vi "RealSense_HelloWorld_PointCloud Plus.vi"() -> ()   [LabVIEW 2023]
doc: "Simple Demo showing how to connect a RealSense Camera to stream COLOR and DEPTH from the stereo camera of a D4xx series camera. \n\nThis expands on the standard sample, by adding \n1. Subsampling for performance enhancement\n2. Collecting time-synched frames, and \n3. Option to remove texture from pointcloud"
uses:
  <vilib>/picture/3D Picture Control/NI_3D Picture Control.lvlib
  <vilib>/Utility/miscctls.llb/LV3DPointTypeDef.ctl
  <vilib>/Utility/miscctls.llb/LVRGBAColorTypeDef.ctl
  <vilib>/picture/3D Picture Control/Object/Create Object (name).vi
panel:
  in  "Display tab":T1(tab)=enum."Color + Depth"
  in  "Sync frames":T2(ring)
  out "Found \nRealSense":bool=TRUE
  out "height":i32=720
  out "width":i32=1280
  out "init results":T3={"camera name"="Intel RealSense 415", "camera S/N"="725112060291", "F/W"="05.08.09.00", "Sensor name"="Stereo Module", "api_version"=20800, "rscontext"=119411024, "device_list"=120905744, "device count"=2, "Dev out"=117239280, "sensor_list"=117821936, "sensor count"=2, "Sensor out"=325562496}
  in  "Select Resolution":u16(ring)=27 items=["424 x 240 @6fps", "424 x 240 @15fps", "424 x 240 @30fps", "424 x 240 @60fps", "424 x 240 @90fps", "480 x 270 @6fps", "480 x 270 @15fps", "480 x 270 @30fps", "480 x 270 @60fps", "480 x 270 @90fps", "640 x 360 @6fps", "640 x 360 @15fps", "640 x 360 @30fps", "640 x 360 @60fps", "640 x 360 @90fps", "640 x 480 @6fps", "640 x 480 @15fps", "640 x 480 @30fps", "640 x 480 @60fps", "640 x 480 @90fps", "848 x 480 @6fps", "848 x 480 @15fps", "848 x 480 @30fps", "848 x 480 @60fps", "848 x 480 @90fps", "1280 x 720 @6fps", "1280 x 720 @15fps", "1280 x 720 @30fps"]
  in  "Sensor index":i32
  in  "Device index":i32
  out "L-R Baseline, mm":sgl=54.83181
  out "fy":sgl=952.6064 format="%#_5g"
  out "fx":sgl=952.6064 format="%#_5g"
  out "ppy":sgl=370.69974 format="%#_5g"
  out "ppx":sgl=634.5728 format="%#_5g"
  in  "Exposure,us":sgl=33000.0
  in  "Autoexposure":bool=TRUE
  in  "Depth Presets":T4(ring)=enum."Face2"
  in  "Color Presets":T5(ring)=enum."DS410 (DS5a) 4"
  in  "Laser on/off":bool=TRUE
  in  "Gain(16-248)":sgl=16.0 min=16 max=248
  in  "Update Presets":bool
  in  "Laser \nPower (mW)":dbl(slide)=155.72448 min=0.0 max=360.0 scale=0.36..360.0
  in  "Range Scale":enum16{"200m", "100m", "60m", "6m", "2m", "1m"}(ring)=enum."6m"
  out "RGB image":picture
  out "Depth map":sgl[][](graph)
  out "3D Picture":refnum<vi>(3d-picture)
  in  "Texture":bool=TRUE
  in  "Time average parameters":T6={"alphaT"=0.3, "deltaDispT(1/32 disp)"=20.0}
  in  "Time Filter":bool=TRUE
  in  "Spatial filter parameters":T7={"alphaXY"=0.5, "deltaDispXY (1/32 disp)"=20.0, "iterations"=2} {"iterations" min=1 max=8; "deltaDispXY (1/32 disp)" min=0.001 max=65000; "alphaXY" min=0.001 max=1}
  in  "Spatial Filter":bool=TRUE
  in  "Persist":bool=TRUE
  out "init error":string="No Error\rNo Error\rNo Error\rNo Error\rNo Error\rNo Error\rNo Error\rNo Error\rNo Error\rNo Error\rNo Error"
  out "Start Error":string="No Error\rNo Error\rNo Error"
  out "Config error":string="No Error\rNo Error"
  out "Close Error":string="No Error\rNo Error\rNo Error\rNo Error"
  out "Time stamp, ms":dbl format="%_10f"
  out "Frame number":u64
  out "Time stamp 2, ms":dbl format="%_10f"
  out "Frame number 2":u64
  out "Timestamp domain":u16(ring) items=["Hardware clock", "System Time", "Count"]
  out "Timestamp domain 2":u16(ring) items=["Hardware clock", "System Time", "Count"]
  out "iteration":i32=357
  in  "stop":bool=TRUE
  # "RealSense Hello World: PointCloud + Post Process"
  # "This demo shows how to connect a RealSense D4xx Stereo Depth Camera, and display the textured PointCloud."
  # "Note; When you change Depth Preset you need to stop and restart for the HDAD settings to take effect.\n\nTry the Color preset called \"Remove IR2\". It will remove the laser projector from the RGB 1280x720 image."
  # "INTRINSICS & EXTRINSICS"
  # "SELECT THE RESOLUTION"
  # "DEPTH MAP"
  # "COLOR"
  # "Changes Color scale for Depth Map."
  # "20-1660000"
  # "3D POINTCLOUD"
  # "Rotate: Drag image\nMove X-Y: HOLD DOWN CTRL while dragging.\nZoom: SHIFT while dragging."
  # "POST PROCESS"
  # "ON\n\nOFF"
  # "Restart to take effect"
  # "Alph can have values from 0 to 1\n1 is zero filtering, and 0 is max filtering."
  # "ERRORS"
  # "If you do not see the Hardware clock then you will need to apply \nWindows fix. See diagram."
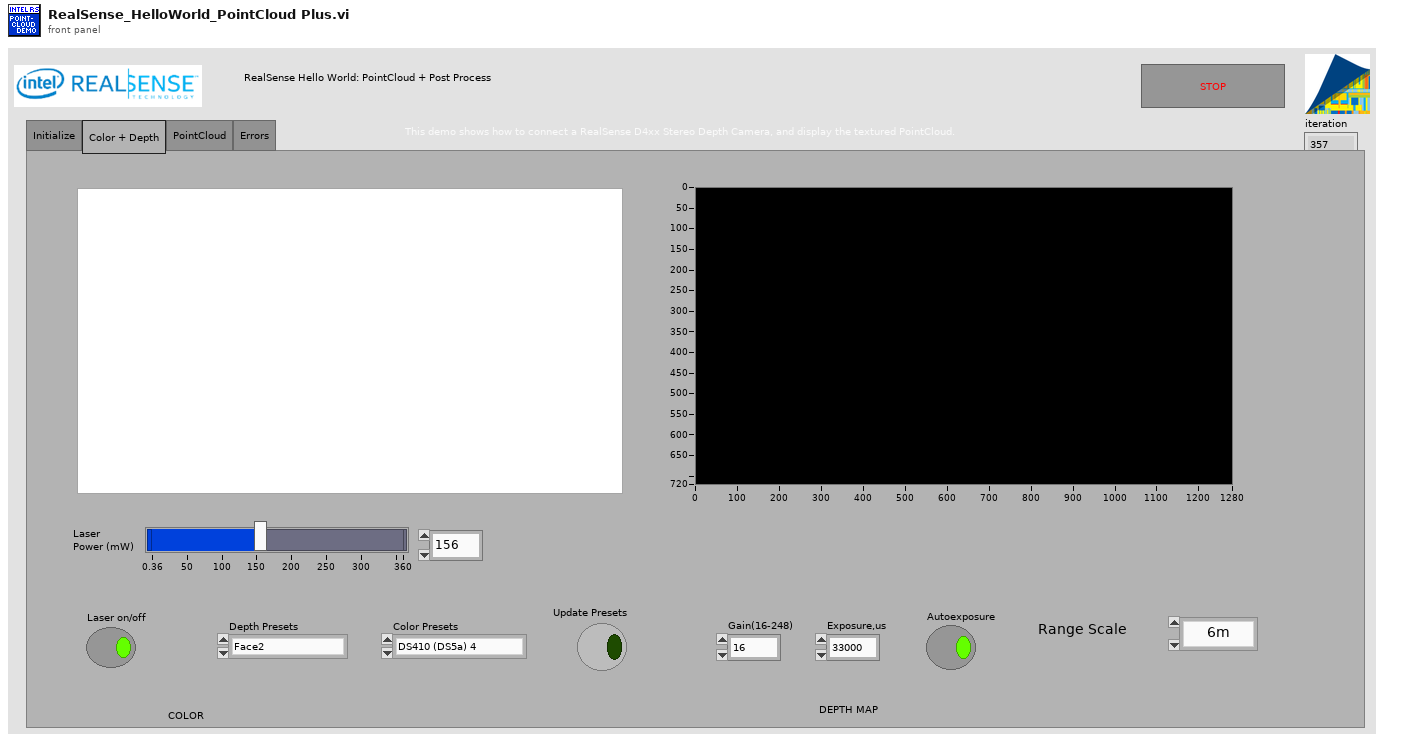
[diagram p1: front panel]
types:
  T1 = enum32{"Initialize", "Color + Depth", "PointCloud", "Errors"}
  T2 = enum16{"Sync on timestamp", "Sync on frame counter"}
  T3 = cluster{"camera name":string, "camera S/N":string, "F/W":string, "Sensor name":string, "api_version":i32, "rscontext":u64, "device_list":u64, "device count":i32, "Dev out":u64, "sensor_list":u64, "sensor count":i32, "Sensor out":u64}
  T4 = enum16{"Custom", "Original", "New Depth 1", "New Depth 2", "Depth Active 1", "Active 3D Scan", "Active Short A", "Active Short C", "Face", "Face2", "Best Box", "High Density", "Medium Density", "High Accuracy", "Hand", "Short Range", "Flat wall", "Load .JSON", "Load .JSON2"}
  T5 = enum16{"Custom", "RS400 (DS5p)", "RS400 (DS5p) 2", "RS400 (DS5p) 3", "RS400 (DS5p) 4", "RS400 (DS5p) 5", "RS410 (DS5a)", "RS410 (DS5a) 2", "DS410 (DS5a) 3", "DS410 (DS5a) 4", "DS410+IR", "DS5LR", "DS5LR-2", "DS5LR no pattern", "RS410 Remove IR", "RS410 Remove IR 2", "DS5micro", "D435"}
  T6 = cluster{"alphaT":sgl, "deltaDispT(1/32 disp)":sgl}
  T7 = cluster{"alphaXY":sgl, "deltaDispXY (1/32 disp)":sgl, "iterations":i32}
  T8 = cluster{"width":i32, "height":i32, "fps":i32, "Profile":u64, "ppx":sgl, "ppy":sgl, "fx":sgl, "fy":sgl, "model":u32}
  T9 = cluster{"Stream type":enum16{"Depth", "Color (ext.)", "Color (left) ", "IR Left", "IR Right", "IR Left (Y16)", "IR Right (Y16)"}, "frame out":u64, "width":i32, "height":i32, "Time stamp":dbl, "Frame number":u64}
  T10 = cluster{"focal length (pixels)":sgl, "baseline, mm":sgl, "z_units":sgl, "Y height":i32, "X width":i32, "Scale":i32, "Color format":enum16{"Monochrome", "RGB internal (RGB)"}}
  T11 = enum16{"Points", "Lines", "Line Strip", "Line Loop", "Triangles", "Triangle Strip", "Triangle Fan", "Quads", "Quad Strip", "Polygon"}
  T12 = enum16{"Overall", "Per Primitive", "Per Vertex", "Binding Off"}
  T13 = typedef "LVRGBAColorTypeDef.ctl" = cluster{"Red":sgl, "Green":sgl, "Blue":sgl, "Alpha":sgl}
  T14 = enum16{"Depth", "Color (ext.)", "Color (left) ", "IR Left", "IR Right", "IR Left (Y16)", "IR Right (Y16)"}
  T15 = cluster{"R":dbl, "G":dbl, "B":dbl, "Alpha":dbl}[]
  T16 = typedef "LV3DPointTypeDef.ctl" = cluster{"X":sgl, "Y":sgl, "Z":sgl}
  T17 = cluster{"Alpha":sgl, "Blue":sgl, "Green":sgl, "Red":sgl}
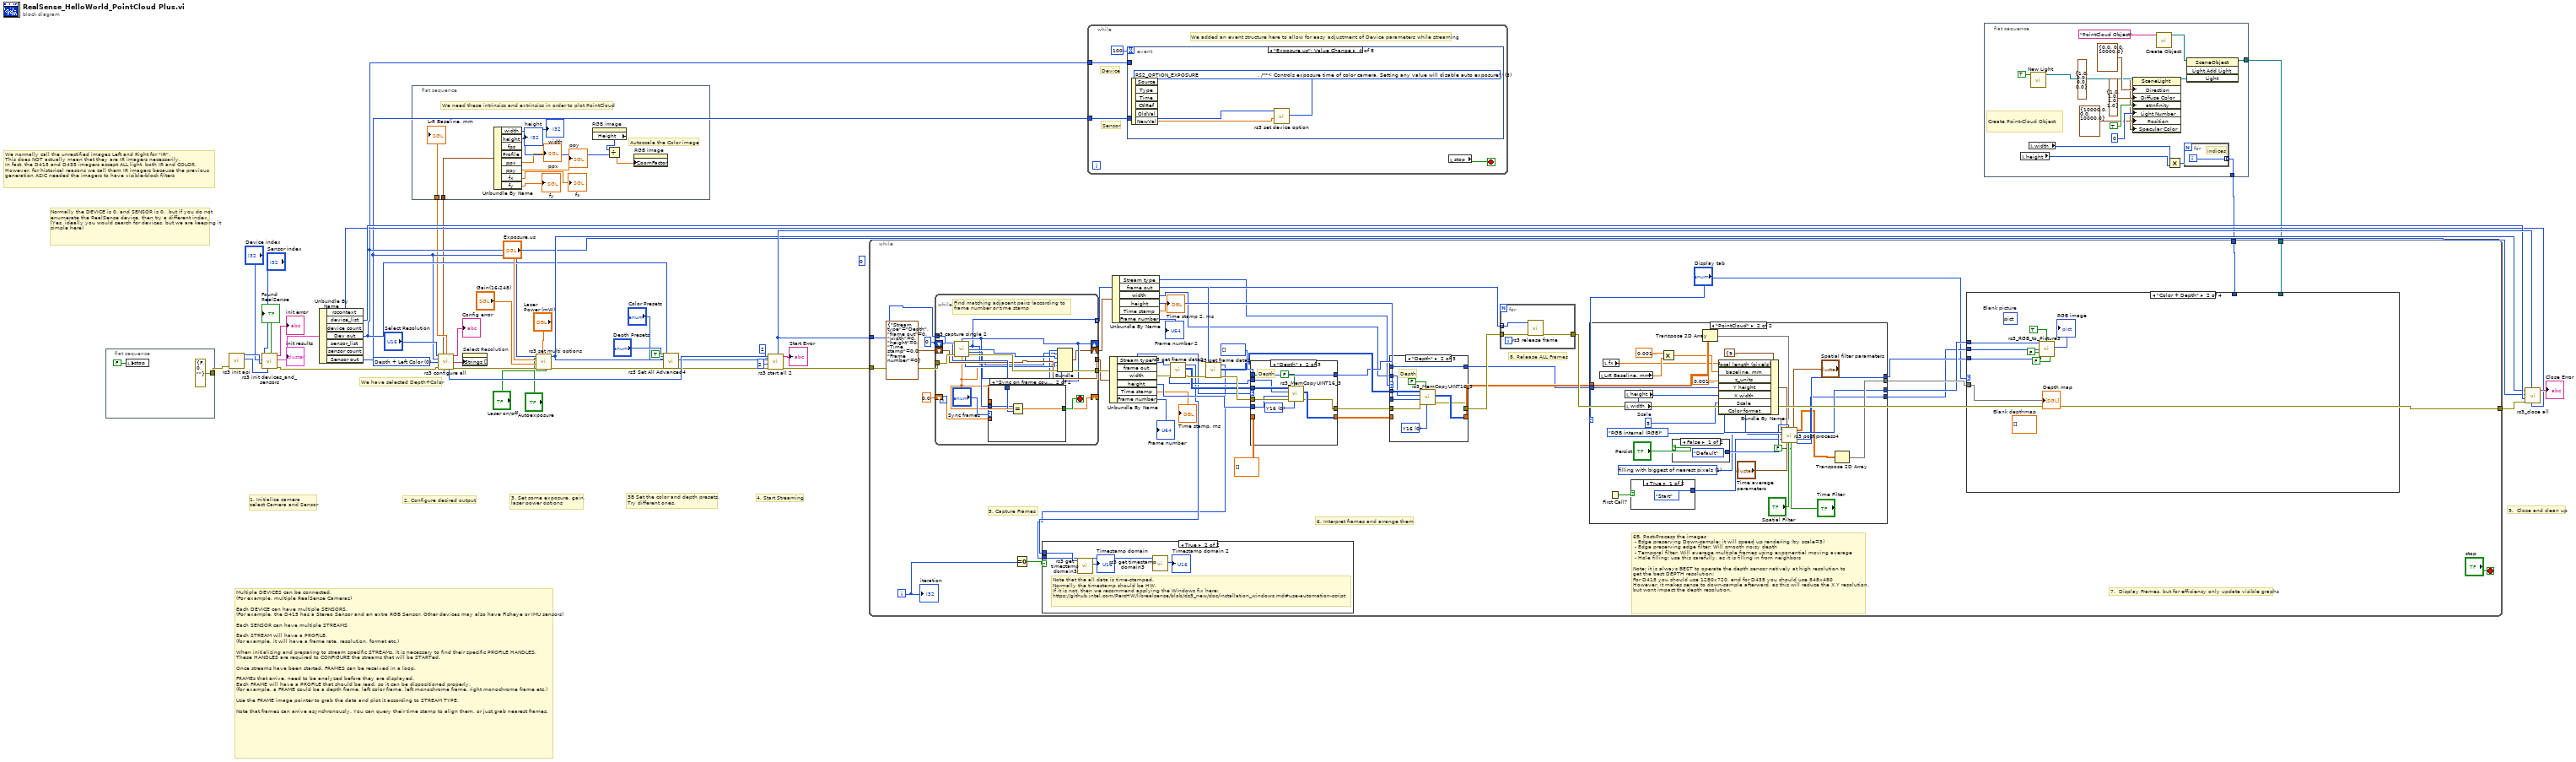
[diagram p0: block diagram]
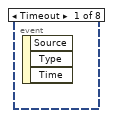
[diagram p2: hidden frame]
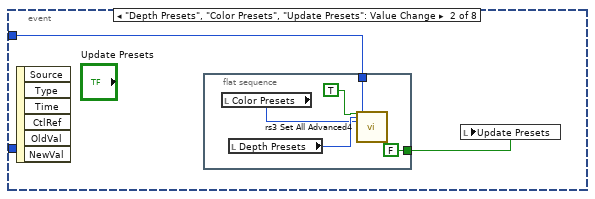
[diagram p3: hidden frame]
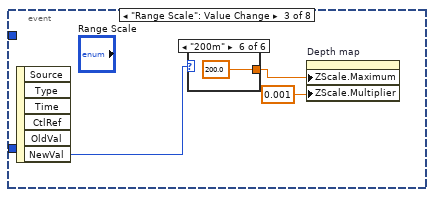
[diagram p4: hidden frame]
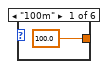
[diagram p5: hidden frame]
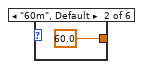
[diagram p6: hidden frame]
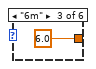
[diagram p7: hidden frame]
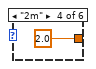
[diagram p8: hidden frame]
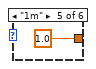
[diagram p9: hidden frame]
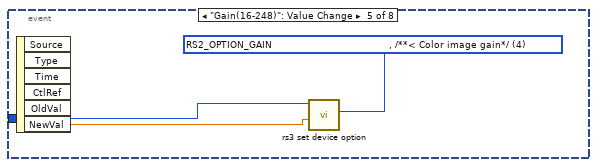
[diagram p10: hidden frame]
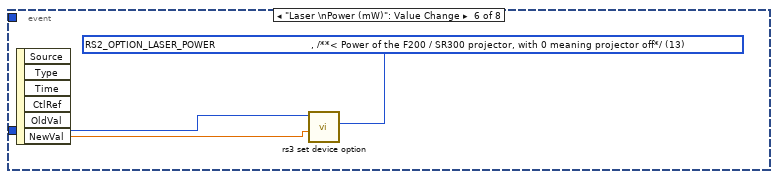
[diagram p11: hidden frame]
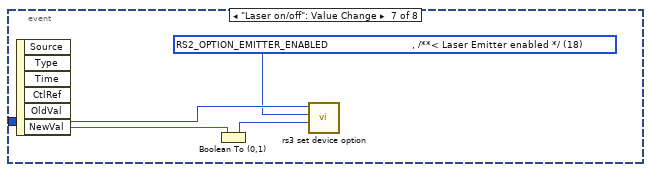
[diagram p12: hidden frame]
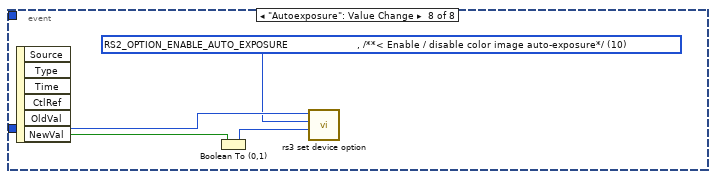
[diagram p13: hidden frame]
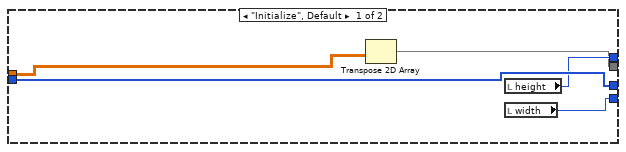
[diagram p14: hidden frame]
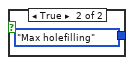
[diagram p15: hidden frame]
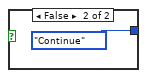
[diagram p16: hidden frame]
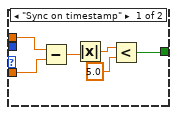
[diagram p18: hidden frame]
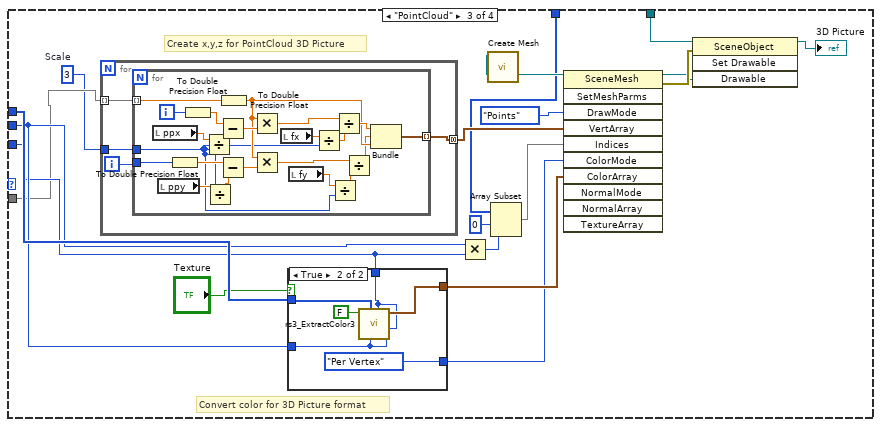
[diagram p20: hidden frame]
diagram:
  (unwired) 0 ("Decimate")
  w29 = u16 0 items=["Depth + Left Color", "Unrectified L + R", "Rectified L + R"] ("Stream selection")
  # "3B Set the color and depth presets.\nTry different ones."
  # "We normally call the unrectified images Left and Right for \"IR\". \nThis does NOT actually mean that they are IR imagers necessarily. \nIn fact, the D415 and D435 imagers accept ALL light, both IR and COLOR.\nHowever, for historical reasons we call them IR imagers because the previous generation ASIC needed the imagers to have visible-block filters"
  # "We have selected Depth+Color"
  # "Normally the DEVICE is 0, and SENSOR is 0,  but if you do not enumerate the RealSense device, then try a different index.\n(Yes, ideally you would search for devices, but we are keeping it simple here)"
  # "Multiple DEVICES can be connected. \n(For example, multiple RealSense Cameras)\n\nEach DEVICE can have multiple SENSORS. \n(For example, the D415 has a Stereo Sensor and an extra RGB Sensor. Other devices may also have Fisheye or IMU sensors) \n\nEach SENSOR can have multiple STREAMS\n\nEach STREAM will have a PROFILE. \n(for example, it will have a frame rate, resolution, format etc.)\n\nWhen initializing and preparing to stream specific STREAMs, it is necessary to find their specific PROFILE HANDLES.\nThese HANDLES are required to CONFIGURE the streams that will be STARTed. \n\nOnce streams have been started, FRAMES can be received in a loop. \n \nFRAMEs that arrive, need to be analyzed before they are displayed. \nEach FRAME will have a PROFILE that should be read, so it can be dispositioned properly.\n(for example, a FRAME could be a depth frame, left color frame, left monochrome frame, right monochrome frame etc.)\n\nUse the FRAME image pointer to grab the data and plot it according to STREAM TYPE.\n\nNote that frames can arrive asynchronously. You can query their time stamp to align them, or just grab nearest frames."
  # "9.  Close and clean up"
  # "4. Start Streaming"
  # "3. Set some exposure, gain, \nlaser power options"
  # "2. Configure desired output"
  # "1. Initialize camera\nselect Camera and Sensor"
  n1 = flat-sequence {
    tunnel: [errorcluster {"status"=FALSE, "code"=0, "source"=""} ("error in")] -> w30
    frame #0 {
      n2 = local write "stop"(FALSE ("stop")) -> ()
    }
  }
  n3 = call "rs3 init api.vi"("error in (no error)"=w30) -> ("rscontext"=w9:u64, "api_version"=w10:i32)  [unwired: 8 in, 1 out]
  n4 = call "rs3 init devices_and_sensors.vi"("rscontext"=w9, "api_version"=w10, "Select Device"="Device index", "Select Sensor"="Sensor index") -> ("error out"=w6:errorcluster, "init results"=w4:T3, "init error"=→"init error":string, "Found RealSense"=→"Found \nRealSense":bool)  [unwired: 1 in, 3 out]
  "init results" <- w4
  n5 = Unbundle By Name(w4) -> ("rscontext"=w35:u64, "device_list"=w36:u64, "Dev out"=w17:u64, "Sensor out"=w16:u64)  [unwired: 3 out]
  n6 = flat-sequence {
    tunnel: w14 -> [w53]
    tunnel: w13 -> [w52]
    frame #0 {
      # "Autoscale the Color image"
      # "We need these intrinsics and extrinsics in order to plot PointCloud"
      n7 = Unbundle By Name(w52) -> ("width"=→"width":i32, "height"=w50:i32, "ppx"=→"ppx":sgl, "ppy"=→"ppy":sgl, "fx"=→"fx":sgl, "fy"=→"fy":sgl)  [unwired: 2 out]
      "height" <- w50
      n8 = property on="RGB image" class="Pict"() -> ("Height"=w51:u32)  [unwired: 2 in, 2 out]
      n9 = Divide(x=w51, y=w50) -> (x/y=w49:dbl)
      n10 = property on="RGB image" class="Pict"("ZoomFactor"=w49) -> ()  [unwired: 2 in, 2 out]
      "L-R Baseline, mm" <- w53
    }
  }
  n11 = call "rs3 configure all.vi"("Select Resolution"="Select Resolution", "Sensor in"=w16, "Stream selection"=w29, "error in (no error)"=w6) -> ("Output stream L"=w13:T8, "config error"=→"Config error":string, "Output stream"=w31:string[], "L-R Baseline, mm"=w14:sgl, "Stream Profile Handles"=w41:u64[], "error out"=w28:errorcluster)  [unwired: 2 in, 4 out]
  n12 = property on="Select Resolution" class="Ring (strict)"("Strings []"=w31) -> ()  [unwired: 2 in, 2 out]
  n13 = call "rs3 set multi options.vi"("laser on/off"="Laser on/off", "autoexposure"="Autoexposure", "Laser power, mW (0-360)"="Laser \nPower (mW)", "error in (no error)"=w28, "Gain(16-248)"="Gain(16-248)", "Exposure, us"="Exposure,us", "Sensor in"=w16) -> ("error out"=w22:errorcluster, "Sensor out"=w27:u64)  [unwired: 2 in, 1 out]
  n14 = call "rs3 Set All Advanced4.vi"("Set Color Corr"=TRUE, "Depth Presets"="Depth Presets", "Color Presets"="Color Presets", "error in (no error)"=w22, "device in"=w17) -> ("error out"=w21:errorcluster)  [unwired: 20 in, 2 out]
  n15 = call "rs3 start all 2.vi"("capacity"=2, "error in (no error)"=w21, "Count of Streams"=2, "Sensor in"=w27, "Stream profile array"=w41) -> ("error out"=w32:errorcluster, "Config Error"=→"Start Error":string, "queue out"=w40:u64)  [unwired: 3 in, 1 out]
  n16 = while {
    tunnel: w40 -> [w94]
    tunnel: w32 -> [w93]
    tunnel: [w73] -> w39
    tunnel: w12 -> [w96]
    tunnel: w11 -> [w95]
    i -> [w65]
    stop <- "stop" stop-if-true
    # "6B. Post-Process the images \n - Edge preserving Down-sample: it will speed up rendering (try scale=3)\n - Edge preserving edge filter: Will smooth noisy depth\n - Temporal filter: Will average multiple frames using exponential moving average\n - Hole filling: use this carefully, as it is filling in from neighbors\n\nNote: it is always BEST to operate the depth sensor natively at high resolution to \nget the best DEPTH resolution: \nFor D415 you should use 1280x720, and for D435 you should use 848x480\nHowever, it makes sense to down-sample afterward, as this will reduce the X,Y resolution, \nbut wont impact the depth resolution."
    # "8. Release ALL Frames"
    # "7.  Display Frames, but for efficiency only update visible graphs"
    # "6. Interpret frames and arrange them"
    # "5. Capture Frames"
    n17 = while {
      tunnel: w94 -> [w159]
      tunnel: [w158] -> w91
      tunnel: w93 -> [w157]
      shift-right: [w150] -> _
      shift-left: u64 0 ("Frame number") -> [w155]
      shift-right: [w149] -> w87
      shift-left: T9 {"Stream type"=enum."Depth", "frame out"=0, "width"=0, "height"=0, "Time stamp"=0.0, "Frame number"=0} -> [w154]
      tunnel: [w154] -> w88
      tunnel: [w148] -> w75 mode=indexing
      shift-right: [w145] -> _
      shift-left: 0.0 ("Time stamp") -> [w146]
      stop <- w156 stop-if-true
      # "Find matching adjacent pairs (according to frame number or time stamp"
      n18 = call "rs3 capture single 2.vi"("queue in"=w159, "error in (no error)"=w157) -> ("Frame number"=w150:u64, "frame out"=w148:u64, "width"=w153:i32, "Stream type"=w151:T14, "Time stamp"=w145:dbl, "height"=w152:i32, "error out"=w158:errorcluster)  [unwired: 3 in, 4 out]
      n19 = case shown="\"Sync on frame counter\"" "Sync frames" {
        tunnel: [w163 w168] -> w156
        tunnel: w155 -> [_ w167]
        tunnel: w150 -> [_ w166]
        tunnel: w146 -> [w165 _]
        tunnel: w145 -> [w164 _]
        frame "Sync on timestamp" {
          n20 = Subtract(x=w164, y=w165) -> (x-y=w162:dbl)
          n21 = Absolute Value(x=w162) -> (abs(x)=w161:dbl)
          n22 = Less?(x=w161, y=5.0) -> (x < y?=w163:bool)
        }
        frame "Sync on frame counter" {
          n23 = Equal?(x=w166, y=w167) -> (x = y?=w168:bool)
        }
      }
      n24 = Bundle("Stream type"=w151, "frame out"=w148, "width"=w153, "height"=w152, "Time stamp"=w145, "Frame number"=w150) -> (w149:T9)  [unwired: 1 in]
    }
    n25 = Equal To 0?(x=w65) -> (x = 0?=w55:bool)
    n26 = Unbundle By Name(w88) -> ("Stream type"=w76:T14, "frame out"=w89:u64, "width"=w78:i32, "height"=w77:i32, "Time stamp"=→"Time stamp, ms":dbl, "Frame number"=→"Frame number":u64)
    n27 = Unbundle By Name(w87) -> ("Stream type"=w57:T14, "frame out"=w86:u64, "width"=w56:i32, "height"=w58:i32, "Time stamp"=→"Time stamp 2, ms":dbl, "Frame number"=→"Frame number 2":u64)
    n28 = call "rs3 get frame data2.vi"("error in (no error)"=w91, "device in"=w89) -> ("error out"=w90:errorcluster, "2D Depth Output"=w81:u16[][], "device out"=w67:u64)  [unwired: 6 in, 1 out]
    n29 = call "rs3 get frame data2.vi"("error in (no error)"=w90, "device in"=w86) -> ("error out"=w83:errorcluster, "2D Depth Output"=w80:u16[][], "device out"=w66:u64)  [unwired: 6 in, 1 out]
    n30 = case shown="True" w55 {
      tunnel: w67 -> [_ w141]
      tunnel: w66 -> [_ w140]
      frame False {
      }
      frame True {
        # "Note that the all data is time-stamped. \nNormally the timestamp should be HW. \nIf it is not, then we recommend applying the Windows fix here:\nhttps://github.intel.com/PercHW/librealsense/blob/ds5_new/doc/installation_windows.md#use-automation-script"
        n31 = call "rs3 get timestamp domain3.vi"("frame in"=w141) -> ("Timestamp domain"=→"Timestamp domain":u16)  [unwired: 7 in, 3 out]
        n32 = call "rs3 get timestamp domain3.vi"("frame in"=w140) -> ("Timestamp domain"=→"Timestamp domain 2":u16)  [unwired: 7 in, 3 out]
      }
    }
    n33 = case shown="\"Depth\"" w76 {
      tunnel: [w250 w259 w268] -> w98
      tunnel: [w252 w260 w266] -> w97
      tunnel: sgl[][] [] ("2D Array Output") -> [w252 _ w266]
      tunnel: u8[] [] ("Output Array") -> [w251 w258 _]
      tunnel: [w251 w258 w267] -> w79
      tunnel: w83 -> [w250 w257 w262]
      tunnel: w81 -> [_ w256 w265]
      tunnel: w78 -> [_ w255 w264]
      tunnel: w77 -> [_ w254 w263]
      frame "Color (ext.)", Default {
      }
      frame "Depth" {
        w261 = u16 0 items=["Y16", "Y8"] ("Image format")
        # "Depth"
        n34 = call "rs3_MemCopyUINT16_3.vi"("Image format"=w261, "Transpose"=FALSE, "error in (no error)"=w257, "Height"=w254, "Width"=w255, "Zimage pointer"=w256) -> ("error out"=w259:errorcluster, "2D Array Output"=w260:u16[][])  [unwired: 4 in]
      }
      frame "Color (left) " {
        # "Color"
        n35 = call "rs3_MemCopyRGB_IR.vi"("Zimage pointer"=w265, "RGB  X, width"=w264, "RGB Y, height"=w263, "Monochrome(T)/Color(F)"=FALSE ("Grey(T)/Color(F)"), "error in (no error)"=w262) -> ("Output Array"=w267:u8[], "error out"=w268:errorcluster)  [unwired: 9 in]
      }
    }
    n36 = case shown="\"Depth\"" w57 {
      tunnel: [w232 w238 w247] -> w74
      tunnel: w98 -> [w232 w239 w248]
      tunnel: w97 -> [w231 _ w245]
      tunnel: [w231 w240 w245] -> w64
      tunnel: [w230 w241 w246] -> w63
      tunnel: w79 -> [w230 w241 _]
      tunnel: w80 -> [_ w236 w244]
      tunnel: w56 -> [_ w235 w242]
      tunnel: w58 -> [_ w234 w243]
      frame "Color (ext.)", Default {
      }
      frame "Depth" {
        w237 = u16 0 items=["Y16", "Y8"] ("Image format")
        # "Depth"
        n37 = call "rs3_MemCopyUINT16_3.vi"("Image format"=w237, "Transpose"=FALSE, "error in (no error)"=w239, "Height"=w234, "Width"=w235, "Zimage pointer"=w236) -> ("error out"=w238:errorcluster, "2D Array Output"=w240:u16[][])  [unwired: 4 in]
      }
      frame "Color (left) " {
        # "Color"
        n38 = call "rs3_MemCopyRGB_IR.vi"("Zimage pointer"=w244, "RGB  X, width"=w242, "RGB Y, height"=w243, "Monochrome(T)/Color(F)"=FALSE ("Grey(T)/Color(F)"), "error in (no error)"=w248) -> ("Output Array"=w246:u8[], "error out"=w247:errorcluster)  [unwired: 9 in]
      }
    }
    n39 = for {
      tunnel: w75 -> [w144] mode=indexing
      tunnel: w74 -> [w143]
      tunnel: [w142] -> w73
      n40 = call "rs3 release frame.vi"("error in (no error)"=w143, "Device"=w144) -> ("error out"=w142:errorcluster)  [unwired: 7 in, 2 out]
    }
    n41 = case shown="\"PointCloud\"" "Display tab" {
      tunnel: w64 -> [w101 w133]
      tunnel: w63 -> [w104 w132]
      tunnel: [w100 w131] -> w62
      tunnel: [w104 w130] -> w61
      tunnel: [w103 w129] -> w60
      tunnel: [w102 w128] -> w59
      frame "Initialize", Default {
        n42 = Transpose 2D Array(2D array=w101) -> (transposed array=w100:sgl[][])
        n43 = local read "height"() -> (w103:i32)
        n44 = local read "width"() -> (w102:i32)
      }
      frame "PointCloud" {
        w115 = 1 items=["filling with left pixel", "filling with biggest of nearest pixels", "filling with smallest of nearest pixels"] ("hole fill algo")
        w127 = 3  # Scale
        n45 = local read "L-R Baseline, mm"() -> (w113:sgl)
        n46 = local read "fx"() -> (w111:sgl)
        n47 = First Call?() -> (First Call?: T/F=w108:bool)
        n48 = local read "height"() -> (w118:i32)
        n49 = local read "width"() -> (w117:i32)
        n50 = case shown="True" w108 {
          tunnel: [enum16{"Start", "Continue", "End", "Do Nothing"}."Start" ("Algo step") enum16{"Start", "Continue", "End", "Do Nothing"}."Continue" ("Algo step")] -> w107
          frame True {
          }
          frame False {
          }
        }
        n51 = Multiply(x=sgl 0.001 ("z_units"), y=w113) -> (x*y=w112:sgl)
        n52 = case shown="False" "Persist" {
          tunnel: [enum16{"Custom", "Default", "Max holefilling"}."Default" ("Temporal persistence \nHole-filling") enum16{"Custom", "Default", "Max holefilling"}."Max holefilling" ("Temporal persistence \nHole-filling")] -> w125
          frame False {
          }
          frame True {
          }
        }
        n53 = Transpose 2D Array(2D array=w133) -> (transposed array=w110:sgl[][])
        n54 = Bundle By Name(cluster=T10 {"focal length (pixels)"=961.0, "baseline, mm"=0.015000001, "z_units"=0.001, "Y height"=720, "X width"=1280, "Scale"=3, "Color format"=enum."RGB internal (RGB)"} ("downsample  parameters"), "focal length (pixels)"=w111, "baseline, mm"=w112, "z_units"=sgl 0.001, "Y height"=w118, "X width"=w117, "Scale"=w127, "Color format"=enum16{"Monochrome", "RGB internal (RGB)"}."RGB internal (RGB)") -> (w120:T10)
        n55 = call "rs3 post process4.vi"("Depth Input"=w110, "Color input"=w132, "hole fill algo"=w115, "Algo step"=w107, "downsample  parameters"=w120, "Time average parameters"="Time average parameters", "Temporal persistence \nHole-filling"=w125, "Spatial Filter"="Spatial Filter", "Time Filter"="Time Filter", "Holefill"=FALSE, "Spatial filter parameters"="Spatial filter parameters") -> ("Depth Output"=w109:sgl[][], "Color output"=w130:u8[], "output width"=w128:i32, "output height"=w129:i32)  [unwired: 4 in, 1 out]
        n56 = Transpose 2D Array(2D array=w109) -> (transposed array=w131:sgl[][])
      }
    }
    n57 = case shown="\"Color + Depth\"" "Display tab" {
      tunnel: w61 -> [_ w173 w195 _]
      tunnel: w62 -> [_ w172 w178 _]
      tunnel: w96 -> [_ _ w187 _]
      tunnel: w95 -> [_ _ w186 _]
      tunnel: w59 -> [_ w171 w180 _]
      tunnel: w60 -> [_ w170 w179 _]
      frame "Initialize", Default {
      }
      frame "Color + Depth" {
        (unwired) sgl[][] []  # Blank depthmap
        (unwired) picture bytes[33]  # Blank picture
        n58 = call "rs3_RGB_to_Picture3.vi"("RGB array"=w173, "Color(T)/Greyscale(F)"=TRUE, "RGB  X, width"=w171, "RGB Y, height"=w170, "AWB"=FALSE, "White Balance"=FALSE) -> ("new picture"=→"RGB image":picture)  [unwired: 8 in, 1 out]
        "Depth map" <- w172
      }
      frame "PointCloud" {
        w177 = 3  # Scale
        # "Convert color for 3D Picture format"
        # "Create x,y,z for PointCloud 3D Picture"
        n59 = for {
          tunnel: w178 -> [w207] mode=indexing
          tunnel: [w206] -> w190 mode=concatenating
          tunnel: w177 -> [w204]
          i -> [w205]
          n60 = for {
            tunnel: w207 -> [w229] mode=indexing
            tunnel: w205 -> [w228]
            tunnel: [w227] -> w206 mode=indexing
            tunnel: w204 -> [w208]
            i -> [w226]
            n61 = local read "ppx"() -> (w216:sgl)
            n62 = local read "ppy"() -> (w214:sgl)
            n63 = To Double Precision Float(number=w228) -> (double precision float=w220:dbl)
            n64 = To Double Precision Float(number=w226) -> (double precision float=w222:dbl)
            n65 = Divide(x=w216, y=w208) -> (x/y=w215:sgl)
            n66 = Divide(x=w214, y=w208) -> (x/y=w213:sgl)
            n67 = Subtract(x=w222, y=w215) -> (x-y=w221:dbl)
            n68 = Subtract(x=w220, y=w213) -> (x-y=w219:dbl)
            n69 = To Double Precision Float(number=w229) -> (double precision float=w218:dbl)
            n70 = Multiply(x=w218, y=w221) -> (x*y=w225:dbl)
            n71 = Multiply(x=w218, y=w219) -> (x*y=w223:dbl)
            n72 = local read "fx"() -> (w212:sgl)
            n73 = local read "fy"() -> (w210:sgl)
            n74 = Divide(x=w212, y=w208) -> (x/y=w211:sgl)
            n75 = Divide(x=w210, y=w208) -> (x/y=w209:sgl)
            n76 = Divide(x=w225, y=w211) -> (x/y=w224:dbl)
            n77 = Divide(x=w223, y=w209) -> (x/y=w217:dbl)
            n78 = Bundle(w224, w217, w218) -> (w227:cluster{dbl, dbl, dbl})  [unwired: 1 in]
          }
        }
        n79 = case shown="True" "Texture" {
          tunnel: w195 -> [_ w203]
          tunnel: [T13[] [{"Red"=1.0, "Green"=1.0, "Blue"=1.0, "Alpha"=0.0}] ("Color Array") w201] -> w189
          tunnel: [T12."Overall" ("Color Binding Mode") T12."Per Vertex" ("Color Binding Mode")] -> w182
          tunnel: w179 -> [_ w198]
          tunnel: w180 -> [_ w199]
          frame False {
          }
          frame True {
            n80 = call "rs3_ExtractColor3.vi"("Depth X"=w199, "Depth Y"=w198, "RGB Y"=w198, "RGB  X"=w199, "24bit Color Array"=w203, "White Balance"=FALSE) -> ("Norm Mesh Color"=w201:T15)  [unwired: 5 in]
          }
        }
        n81 = Multiply(x=w180, y=w179) -> (x*y=w183:i32)
        n82 = call <vilib>:"Create Mesh.vi"() -> ("New Mesh Refnum"=w192:refnum<vi>)  [unwired: 10 in, 1 out]
        n83 = Array Subset(array=w186, index=0, length=w183) -> (w185:i32[])
        n84 = invoke class="SceneMesh" method="SetMeshParms"(reference=w192, "DrawMode"=T11."Points" ("Draw Mode"), "VertArray"=w190, "Indices"=w185, "ColorMode"=w182, "ColorArray"=w189) -> (reference out=w193:refnum<vi>, error out=w194:errorcluster)  [unwired: 5 in, 9 out]
        n85 = invoke class="SceneObject" method="Set Drawable"(reference=w187, error in=w194, "Drawable"=w193) -> (reference out=→"3D Picture":refnum<vi>)  [unwired: 1 in, 3 out]
      }
      frame "Errors" {
      }
    }
    "iteration" <- w65
  }
  n86 = while {
    tunnel: w17 -> [w272]
    tunnel: w16 -> [w271]
    stop <- w273 stop-if-true
    # "Sensor"
    # "Device"
    # "We added an event structure here to allow for easy adjustment of Device parameters while streaming"
    n87 = event shown="[3] \"Exposure,us\": Value Change" {
      selector: _ -> [_ _ _ _ _ _ _ _]
      dyn-events: _ -> [_ _ _ _ _ _ _ _]
      timeout: 100 -> [_ _ _ _ _ _ _ _]
      tunnel: w272 -> [_ w275 _ _ _ _ _ _]
      tunnel: w271 -> [_ _ _ w292 w295 w298 w302 w306]
      event Timeout {
        n88 = event-data() -> ()  [unwired: 1 in, 3 out]
      }
      event "Depth Presets", "Color Presets", "Update Presets": Value Change {
        n89 = event-data() -> ()  [unwired: 1 in, 6 out]
        n90 = flat-sequence {
          tunnel: w275 -> [w277]
          tunnel: [FALSE ("Update Presets")] -> w274
          frame #0 {
            n91 = local read "Color Presets"() -> (w279:T5)
            n92 = local read "Depth Presets"() -> (w280:T4)
            n93 = call "rs3 Set All Advanced4.vi"("Set Color Corr"=TRUE, "Depth Presets"=w280, "Color Presets"=w279, "device in"=w277) -> ()  [unwired: 21 in, 3 out]
          }
        }
        n94 = local write "Update Presets"(w274) -> ()
      }
      event "Range Scale": Value Change {
        n95 = event-data() -> ("NewVal"=w282:enum16{"200m", "100m", "60m", "6m", "2m", "1m"})  [unwired: 1 in, 5 out]
        n96 = case shown="\"200m\"" w282 {
          tunnel: [100.0 ("Z Scale.Offset and Multiplier:Multiplier") 60.0 ("Z Scale.Offset and Multiplier:Multiplier") 6.0 ("Z Scale.Offset and Multiplier:Multiplier") 2.0 ("Z Scale.Offset and Multiplier:Multiplier") 1.0 ("Z Scale.Offset and Multiplier:Multiplier") 200.0 ("Z Scale.Offset and Multiplier:Multiplier")] -> w281
          frame "100m" {
          }
          frame "60m", Default {
          }
          frame "6m" {
          }
          frame "2m" {
          }
          frame "1m" {
          }
          frame "200m" {
          }
        }
        n97 = property on="Depth map" class="IntGraph (strict)"("ZScale.Maximum"=w281, "ZScale.Multiplier"=0.001 ("Z Scale.Offset and Multiplier:Multiplier")) -> ()  [unwired: 2 in, 2 out]
      }
      event "Exposure,us": Value Change {
        w290 = u16 3 items=["    RS2_OPTION_BACKLIGHT_COMPENSATION                     , /**< Enable / disable color backlight compensation*/", "    RS2_OPTION_BRIGHTNESS                                 , /**< Color image brightness*/", "    RS2_OPTION_CONTRAST                                   , /**< Color image contrast*/", "    RS2_OPTION_EXPOSURE                                   , /**< Controls exposure time of color camera. Setting any value will disable auto exposure*/", "    RS2_OPTION_GAIN                                       , /**< Color image gain*/", "    RS2_OPTION_GAMMA                                      , /**< Color image gamma setting*/", "    RS2_OPTION_HUE                                        , /**< Color image hue*/", "    RS2_OPTION_SATURATION                                 , /**< Color image saturation setting*/", "    RS2_OPTION_SHARPNESS                                  , /**< Color image sharpness setting*/", "    RS2_OPTION_WHITE_BALANCE                              , /**< Controls white balance of color image. Setting any value will disable auto white balance*/", "    RS2_OPTION_ENABLE_AUTO_EXPOSURE                       , /**< Enable / disable color image auto-exposure*/", "    RS2_OPTION_ENABLE_AUTO_WHITE_BALANCE                  , /**< Enable / disable color image auto-white-balance*/", "    RS2_OPTION_VISUAL_PRESET                              , /**< Provide access to several recommend sets of option presets for the depth camera */", "    RS2_OPTION_LASER_POWER                                , /**< Power of the F200 / SR300 projector, with 0 meaning projector off*/", "    RS2_OPTION_ACCURACY                                   , /**< Set the number of patterns projected per frame. The higher the accuracy value the more patterns projected. Increasing the number of patterns help to achieve better accuracy. Note that this c", "    RS2_OPTION_MOTION_RANGE                               , /**< Motion vs. Range trade-off, with lower values allowing for better motion sensitivity and higher values allowing for better depth range*/", "    RS2_OPTION_FILTER_OPTION                              , /**< Set the filter to apply to each depth frame. Each one of the filter is optimized per the application requirements*/", "    RS2_OPTION_CONFIDENCE_THRESHOLD                       , /**< The confidence level threshold used by the Depth algorithm pipe to set whether a pixel will get a valid range or will be marked with invalid range*/", "    RS2_OPTION_EMITTER_ENABLED                            , /**< Laser Emitter enabled */", "    RS2_OPTION_FRAMES_QUEUE_SIZE                          , /**< Number of frames the user is allowed to keep per stream. Trying to hold-on to more frames will cause frame-drops.*/", "    RS2_OPTION_TOTAL_FRAME_DROPS                          , /**< Total number of detected frame drops from all streams */", "    RS2_OPTION_AUTO_EXPOSURE_MODE                         , /**< Auto-Exposure modes: Static, Anti-Flicker and Hybrid */", "    RS2_OPTION_POWER_LINE_FREQUENCY                       , /**< Power Line Frequency control for anti-flickering Off/50Hz/60Hz/Auto */", "    RS2_OPTION_ASIC_TEMPERATURE                           , /**< Current Asic Temperature */", "    RS2_OPTION_ERROR_POLLING_ENABLED                      , /**< disable error handling */", "    RS2_OPTION_PROJECTOR_TEMPERATURE                      , /**< Current Projector Temperature */", "    RS2_OPTION_OUTPUT_TRIGGER_ENABLED                     , /**< Enable / disable trigger to be outputed from the camera to any external device on every depth frame */", "    RS2_OPTION_MOTION_MODULE_TEMPERATURE                  , /**< Current Motion-Module Temperature */", "    RS2_OPTION_DEPTH_UNITS                                , /**< Number of meters represented by a single depth unit */", "    RS2_OPTION_ENABLE_MOTION_CORRECTION                   , /**< Enable/Disable automatic correction of the motion data */", "    RS2_OPTION_AUTO_EXPOSURE_PRIORITY                     , /**< Allows sensor to dynamically ajust the frame rate depending on lighting conditions */", "    RS2_OPTION_COUNT                                      , /**< Number of enumeration values. Not a valid input: intended to be used in for-loops. */"] ("RS Option")
        n98 = event-data() -> ("NewVal"=w291:sgl)  [unwired: 1 in, 5 out]
        n99 = call "rs3 set device option.vi"("value"=w291, "RS Option"=w290, "Sensor in"=w292) -> ()  [unwired: 6 in, 3 out]
      }
      event "Gain(16-248)": Value Change {
        w293 = u16 4 items=["    RS2_OPTION_BACKLIGHT_COMPENSATION                     , /**< Enable / disable color backlight compensation*/", "    RS2_OPTION_BRIGHTNESS                                 , /**< Color image brightness*/", "    RS2_OPTION_CONTRAST                                   , /**< Color image contrast*/", "    RS2_OPTION_EXPOSURE                                   , /**< Controls exposure time of color camera. Setting any value will disable auto exposure*/", "    RS2_OPTION_GAIN                                       , /**< Color image gain*/", "    RS2_OPTION_GAMMA                                      , /**< Color image gamma setting*/", "    RS2_OPTION_HUE                                        , /**< Color image hue*/", "    RS2_OPTION_SATURATION                                 , /**< Color image saturation setting*/", "    RS2_OPTION_SHARPNESS                                  , /**< Color image sharpness setting*/", "    RS2_OPTION_WHITE_BALANCE                              , /**< Controls white balance of color image. Setting any value will disable auto white balance*/", "    RS2_OPTION_ENABLE_AUTO_EXPOSURE                       , /**< Enable / disable color image auto-exposure*/", "    RS2_OPTION_ENABLE_AUTO_WHITE_BALANCE                  , /**< Enable / disable color image auto-white-balance*/", "    RS2_OPTION_VISUAL_PRESET                              , /**< Provide access to several recommend sets of option presets for the depth camera */", "    RS2_OPTION_LASER_POWER                                , /**< Power of the F200 / SR300 projector, with 0 meaning projector off*/", "    RS2_OPTION_ACCURACY                                   , /**< Set the number of patterns projected per frame. The higher the accuracy value the more patterns projected. Increasing the number of patterns help to achieve better accuracy. Note that this c", "    RS2_OPTION_MOTION_RANGE                               , /**< Motion vs. Range trade-off, with lower values allowing for better motion sensitivity and higher values allowing for better depth range*/", "    RS2_OPTION_FILTER_OPTION                              , /**< Set the filter to apply to each depth frame. Each one of the filter is optimized per the application requirements*/", "    RS2_OPTION_CONFIDENCE_THRESHOLD                       , /**< The confidence level threshold used by the Depth algorithm pipe to set whether a pixel will get a valid range or will be marked with invalid range*/", "    RS2_OPTION_EMITTER_ENABLED                            , /**< Laser Emitter enabled */", "    RS2_OPTION_FRAMES_QUEUE_SIZE                          , /**< Number of frames the user is allowed to keep per stream. Trying to hold-on to more frames will cause frame-drops.*/", "    RS2_OPTION_TOTAL_FRAME_DROPS                          , /**< Total number of detected frame drops from all streams */", "    RS2_OPTION_AUTO_EXPOSURE_MODE                         , /**< Auto-Exposure modes: Static, Anti-Flicker and Hybrid */", "    RS2_OPTION_POWER_LINE_FREQUENCY                       , /**< Power Line Frequency control for anti-flickering Off/50Hz/60Hz/Auto */", "    RS2_OPTION_ASIC_TEMPERATURE                           , /**< Current Asic Temperature */", "    RS2_OPTION_ERROR_POLLING_ENABLED                      , /**< disable error handling */", "    RS2_OPTION_PROJECTOR_TEMPERATURE                      , /**< Current Projector Temperature */", "    RS2_OPTION_OUTPUT_TRIGGER_ENABLED                     , /**< Enable / disable trigger to be outputed from the camera to any external device on every depth frame */", "    RS2_OPTION_MOTION_MODULE_TEMPERATURE                  , /**< Current Motion-Module Temperature */", "    RS2_OPTION_DEPTH_UNITS                                , /**< Number of meters represented by a single depth unit */", "    RS2_OPTION_ENABLE_MOTION_CORRECTION                   , /**< Enable/Disable automatic correction of the motion data */", "    RS2_OPTION_AUTO_EXPOSURE_PRIORITY                     , /**< Allows sensor to dynamically ajust the frame rate depending on lighting conditions */", "    RS2_OPTION_COUNT                                      , /**< Number of enumeration values. Not a valid input: intended to be used in for-loops. */"] ("RS Option")
        n100 = event-data() -> ("NewVal"=w294:sgl)  [unwired: 1 in, 5 out]
        n101 = call "rs3 set device option.vi"("value"=w294, "RS Option"=w293, "Sensor in"=w295) -> ()  [unwired: 6 in, 3 out]
      }
      event "Laser \nPower (mW)": Value Change {
        w296 = u16 13 items=["    RS2_OPTION_BACKLIGHT_COMPENSATION                     , /**< Enable / disable color backlight compensation*/", "    RS2_OPTION_BRIGHTNESS                                 , /**< Color image brightness*/", "    RS2_OPTION_CONTRAST                                   , /**< Color image contrast*/", "    RS2_OPTION_EXPOSURE                                   , /**< Controls exposure time of color camera. Setting any value will disable auto exposure*/", "    RS2_OPTION_GAIN                                       , /**< Color image gain*/", "    RS2_OPTION_GAMMA                                      , /**< Color image gamma setting*/", "    RS2_OPTION_HUE                                        , /**< Color image hue*/", "    RS2_OPTION_SATURATION                                 , /**< Color image saturation setting*/", "    RS2_OPTION_SHARPNESS                                  , /**< Color image sharpness setting*/", "    RS2_OPTION_WHITE_BALANCE                              , /**< Controls white balance of color image. Setting any value will disable auto white balance*/", "    RS2_OPTION_ENABLE_AUTO_EXPOSURE                       , /**< Enable / disable color image auto-exposure*/", "    RS2_OPTION_ENABLE_AUTO_WHITE_BALANCE                  , /**< Enable / disable color image auto-white-balance*/", "    RS2_OPTION_VISUAL_PRESET                              , /**< Provide access to several recommend sets of option presets for the depth camera */", "    RS2_OPTION_LASER_POWER                                , /**< Power of the F200 / SR300 projector, with 0 meaning projector off*/", "    RS2_OPTION_ACCURACY                                   , /**< Set the number of patterns projected per frame. The higher the accuracy value the more patterns projected. Increasing the number of patterns help to achieve better accuracy. Note that this c", "    RS2_OPTION_MOTION_RANGE                               , /**< Motion vs. Range trade-off, with lower values allowing for better motion sensitivity and higher values allowing for better depth range*/", "    RS2_OPTION_FILTER_OPTION                              , /**< Set the filter to apply to each depth frame. Each one of the filter is optimized per the application requirements*/", "    RS2_OPTION_CONFIDENCE_THRESHOLD                       , /**< The confidence level threshold used by the Depth algorithm pipe to set whether a pixel will get a valid range or will be marked with invalid range*/", "    RS2_OPTION_EMITTER_ENABLED                            , /**< Laser Emitter enabled */", "    RS2_OPTION_FRAMES_QUEUE_SIZE                          , /**< Number of frames the user is allowed to keep per stream. Trying to hold-on to more frames will cause frame-drops.*/", "    RS2_OPTION_TOTAL_FRAME_DROPS                          , /**< Total number of detected frame drops from all streams */", "    RS2_OPTION_AUTO_EXPOSURE_MODE                         , /**< Auto-Exposure modes: Static, Anti-Flicker and Hybrid */", "    RS2_OPTION_POWER_LINE_FREQUENCY                       , /**< Power Line Frequency control for anti-flickering Off/50Hz/60Hz/Auto */", "    RS2_OPTION_ASIC_TEMPERATURE                           , /**< Current Asic Temperature */", "    RS2_OPTION_ERROR_POLLING_ENABLED                      , /**< disable error handling */", "    RS2_OPTION_PROJECTOR_TEMPERATURE                      , /**< Current Projector Temperature */", "    RS2_OPTION_OUTPUT_TRIGGER_ENABLED                     , /**< Enable / disable trigger to be outputed from the camera to any external device on every depth frame */", "    RS2_OPTION_MOTION_MODULE_TEMPERATURE                  , /**< Current Motion-Module Temperature */", "    RS2_OPTION_DEPTH_UNITS                                , /**< Number of meters represented by a single depth unit */", "    RS2_OPTION_ENABLE_MOTION_CORRECTION                   , /**< Enable/Disable automatic correction of the motion data */", "    RS2_OPTION_AUTO_EXPOSURE_PRIORITY                     , /**< Allows sensor to dynamically ajust the frame rate depending on lighting conditions */", "    RS2_OPTION_COUNT                                      , /**< Number of enumeration values. Not a valid input: intended to be used in for-loops. */"] ("RS Option")
        n102 = event-data() -> ("NewVal"=w297:dbl)  [unwired: 1 in, 5 out]
        n103 = call "rs3 set device option.vi"("value"=w297, "RS Option"=w296, "Sensor in"=w298) -> ()  [unwired: 6 in, 3 out]
      }
      event "Laser on/off": Value Change {
        w301 = u16 18 items=["    RS2_OPTION_BACKLIGHT_COMPENSATION                     , /**< Enable / disable color backlight compensation*/", "    RS2_OPTION_BRIGHTNESS                                 , /**< Color image brightness*/", "    RS2_OPTION_CONTRAST                                   , /**< Color image contrast*/", "    RS2_OPTION_EXPOSURE                                   , /**< Controls exposure time of color camera. Setting any value will disable auto exposure*/", "    RS2_OPTION_GAIN                                       , /**< Color image gain*/", "    RS2_OPTION_GAMMA                                      , /**< Color image gamma setting*/", "    RS2_OPTION_HUE                                        , /**< Color image hue*/", "    RS2_OPTION_SATURATION                                 , /**< Color image saturation setting*/", "    RS2_OPTION_SHARPNESS                                  , /**< Color image sharpness setting*/", "    RS2_OPTION_WHITE_BALANCE                              , /**< Controls white balance of color image. Setting any value will disable auto white balance*/", "    RS2_OPTION_ENABLE_AUTO_EXPOSURE                       , /**< Enable / disable color image auto-exposure*/", "    RS2_OPTION_ENABLE_AUTO_WHITE_BALANCE                  , /**< Enable / disable color image auto-white-balance*/", "    RS2_OPTION_VISUAL_PRESET                              , /**< Provide access to several recommend sets of option presets for the depth camera */", "    RS2_OPTION_LASER_POWER                                , /**< Power of the F200 / SR300 projector, with 0 meaning projector off*/", "    RS2_OPTION_ACCURACY                                   , /**< Set the number of patterns projected per frame. The higher the accuracy value the more patterns projected. Increasing the number of patterns help to achieve better accuracy. Note that this c", "    RS2_OPTION_MOTION_RANGE                               , /**< Motion vs. Range trade-off, with lower values allowing for better motion sensitivity and higher values allowing for better depth range*/", "    RS2_OPTION_FILTER_OPTION                              , /**< Set the filter to apply to each depth frame. Each one of the filter is optimized per the application requirements*/", "    RS2_OPTION_CONFIDENCE_THRESHOLD                       , /**< The confidence level threshold used by the Depth algorithm pipe to set whether a pixel will get a valid range or will be marked with invalid range*/", "    RS2_OPTION_EMITTER_ENABLED                            , /**< Laser Emitter enabled */", "    RS2_OPTION_FRAMES_QUEUE_SIZE                          , /**< Number of frames the user is allowed to keep per stream. Trying to hold-on to more frames will cause frame-drops.*/", "    RS2_OPTION_TOTAL_FRAME_DROPS                          , /**< Total number of detected frame drops from all streams */", "    RS2_OPTION_AUTO_EXPOSURE_MODE                         , /**< Auto-Exposure modes: Static, Anti-Flicker and Hybrid */", "    RS2_OPTION_POWER_LINE_FREQUENCY                       , /**< Power Line Frequency control for anti-flickering Off/50Hz/60Hz/Auto */", "    RS2_OPTION_ASIC_TEMPERATURE                           , /**< Current Asic Temperature */", "    RS2_OPTION_ERROR_POLLING_ENABLED                      , /**< disable error handling */", "    RS2_OPTION_PROJECTOR_TEMPERATURE                      , /**< Current Projector Temperature */", "    RS2_OPTION_OUTPUT_TRIGGER_ENABLED                     , /**< Enable / disable trigger to be outputed from the camera to any external device on every depth frame */", "    RS2_OPTION_MOTION_MODULE_TEMPERATURE                  , /**< Current Motion-Module Temperature */", "    RS2_OPTION_DEPTH_UNITS                                , /**< Number of meters represented by a single depth unit */", "    RS2_OPTION_ENABLE_MOTION_CORRECTION                   , /**< Enable/Disable automatic correction of the motion data */", "    RS2_OPTION_AUTO_EXPOSURE_PRIORITY                     , /**< Allows sensor to dynamically ajust the frame rate depending on lighting conditions */", "    RS2_OPTION_COUNT                                      , /**< Number of enumeration values. Not a valid input: intended to be used in for-loops. */"] ("RS Option")
        n104 = event-data() -> ("NewVal"=w300:bool)  [unwired: 1 in, 5 out]
        n105 = Boolean To (0,1)(Boolean=w300) -> (0, 1=w299:i16)
        n106 = call "rs3 set device option.vi"("value"=w299, "RS Option"=w301, "Sensor in"=w302) -> ()  [unwired: 6 in, 3 out]
      }
      event "Autoexposure": Value Change {
        w305 = u16 10 items=["    RS2_OPTION_BACKLIGHT_COMPENSATION                     , /**< Enable / disable color backlight compensation*/", "    RS2_OPTION_BRIGHTNESS                                 , /**< Color image brightness*/", "    RS2_OPTION_CONTRAST                                   , /**< Color image contrast*/", "    RS2_OPTION_EXPOSURE                                   , /**< Controls exposure time of color camera. Setting any value will disable auto exposure*/", "    RS2_OPTION_GAIN                                       , /**< Color image gain*/", "    RS2_OPTION_GAMMA                                      , /**< Color image gamma setting*/", "    RS2_OPTION_HUE                                        , /**< Color image hue*/", "    RS2_OPTION_SATURATION                                 , /**< Color image saturation setting*/", "    RS2_OPTION_SHARPNESS                                  , /**< Color image sharpness setting*/", "    RS2_OPTION_WHITE_BALANCE                              , /**< Controls white balance of color image. Setting any value will disable auto white balance*/", "    RS2_OPTION_ENABLE_AUTO_EXPOSURE                       , /**< Enable / disable color image auto-exposure*/", "    RS2_OPTION_ENABLE_AUTO_WHITE_BALANCE                  , /**< Enable / disable color image auto-white-balance*/", "    RS2_OPTION_VISUAL_PRESET                              , /**< Provide access to several recommend sets of option presets for the depth camera */", "    RS2_OPTION_LASER_POWER                                , /**< Power of the F200 / SR300 projector, with 0 meaning projector off*/", "    RS2_OPTION_ACCURACY                                   , /**< Set the number of patterns projected per frame. The higher the accuracy value the more patterns projected. Increasing the number of patterns help to achieve better accuracy. Note that this c", "    RS2_OPTION_MOTION_RANGE                               , /**< Motion vs. Range trade-off, with lower values allowing for better motion sensitivity and higher values allowing for better depth range*/", "    RS2_OPTION_FILTER_OPTION                              , /**< Set the filter to apply to each depth frame. Each one of the filter is optimized per the application requirements*/", "    RS2_OPTION_CONFIDENCE_THRESHOLD                       , /**< The confidence level threshold used by the Depth algorithm pipe to set whether a pixel will get a valid range or will be marked with invalid range*/", "    RS2_OPTION_EMITTER_ENABLED                            , /**< Laser Emitter enabled */", "    RS2_OPTION_FRAMES_QUEUE_SIZE                          , /**< Number of frames the user is allowed to keep per stream. Trying to hold-on to more frames will cause frame-drops.*/", "    RS2_OPTION_TOTAL_FRAME_DROPS                          , /**< Total number of detected frame drops from all streams */", "    RS2_OPTION_AUTO_EXPOSURE_MODE                         , /**< Auto-Exposure modes: Static, Anti-Flicker and Hybrid */", "    RS2_OPTION_POWER_LINE_FREQUENCY                       , /**< Power Line Frequency control for anti-flickering Off/50Hz/60Hz/Auto */", "    RS2_OPTION_ASIC_TEMPERATURE                           , /**< Current Asic Temperature */", "    RS2_OPTION_ERROR_POLLING_ENABLED                      , /**< disable error handling */", "    RS2_OPTION_PROJECTOR_TEMPERATURE                      , /**< Current Projector Temperature */", "    RS2_OPTION_OUTPUT_TRIGGER_ENABLED                     , /**< Enable / disable trigger to be outputed from the camera to any external device on every depth frame */", "    RS2_OPTION_MOTION_MODULE_TEMPERATURE                  , /**< Current Motion-Module Temperature */", "    RS2_OPTION_DEPTH_UNITS                                , /**< Number of meters represented by a single depth unit */", "    RS2_OPTION_ENABLE_MOTION_CORRECTION                   , /**< Enable/Disable automatic correction of the motion data */", "    RS2_OPTION_AUTO_EXPOSURE_PRIORITY                     , /**< Allows sensor to dynamically ajust the frame rate depending on lighting conditions */", "    RS2_OPTION_COUNT                                      , /**< Number of enumeration values. Not a valid input: intended to be used in for-loops. */"] ("RS Option")
        n107 = event-data() -> ("NewVal"=w304:bool)  [unwired: 1 in, 5 out]
        n108 = Boolean To (0,1)(Boolean=w304) -> (0, 1=w303:i16)
        n109 = call "rs3 set device option.vi"("value"=w303, "RS Option"=w305, "Sensor in"=w306) -> ()  [unwired: 6 in, 3 out]
      }
    }
    n110 = local read "stop"() -> (w273:bool)
  }
  n111 = flat-sequence {
    tunnel: [w311] -> w12
    tunnel: [w307] -> w11
    frame #0 {
      # "Create Point-Cloud Object"
      n112 = local read "height"() -> (w308:i32)
      n113 = local read "width"() -> (w309:i32)
      n114 = call <vilib>:"New Light.vi"("At Infinity"=TRUE) -> ("New Light Refnum"=w319:refnum<vi>)  [unwired: 2 in, 8 out]
      n115 = property class="SceneLight"(reference=w319, "Direction"=cluster{"X":sgl, "Y":sgl, "Z":sgl} {"X"=0.0, "Y"=0.0, "Z"=10000.0}, "Diffuse Color"=T17 {"Alpha"=1.0, "Blue"=1.0, "Green"=1.0, "Red"=1.0}, "atInfinity"=TRUE ("At Infinity"), "Light Number"=0, "Position"=T16 {"X"=10000.0, "Y"=0.0, "Z"=10000.0}, "Specular Color"=T13 {"Red"=1.0, "Green"=0.0, "Blue"=0.0, "Alpha"=0.0}) -> (reference out=w316:refnum<vi>)  [unwired: 1 in, 1 out]
      n116 = call-poly <vilib>:"Create Object.vi"("Name"="PointCloud Object") -> ("Scene:New Object"=w318:refnum<vi>)  [unwired: 9 in, 1 out]
      n117 = Multiply(x=w309, y=w308) -> (x*y=w310:i32)
      n118 = for {
        N: w310 -> [_]
        tunnel: [w323] -> w307 mode=indexing
        i -> [w323]
        # "indices"
      }
      n119 = invoke class="SceneObject" method="Light.Add Light"(reference=w318, "Light"=w316) -> (reference out=w311:refnum<vi>)  [unwired: 2 in, 3 out]
    }
  }
  n120 = call "rs3_close all.vi"("rscontext"=w35, "queue in"=w40, "error in (no error)"=w39, "device_list"=w36, "Dev in"=w17, "Sensor in"=w27) -> ("Close Error"=→"Close Error":string)  [unwired: 4 in, 1 out]
